vi "Global Event Filter Example - Filter From Subscriber.vi"() -> ()   [LabVIEW 2017]
uses:
  user.lib/_NEVSTOP/Communicable State Machine(CSM)/_Support/Typedef/_CSM_GlobalLog Filter Rules - v1.0.ctl
  user.lib/_NEVSTOP/Communicable State Machine(CSM)/_Support/Typedef/_CSM_GlobalLog_MSG_TYPE.ctl
  user.lib/_NEVSTOP/Communicable State Machine(CSM)/_Support/Typedef/_CSM_GlobalLog_STATE_TYPE.ctl
  user.lib/_NEVSTOP/Communicable State Machine(CSM)/_Support/Typedef/_CSM_GlobalLog_MSG.ctl
  user.lib/_NEVSTOP/Communicable State Machine(CSM)/_Support/Typedef/_CSM_Response Source Message.ctl
  user.lib/_NEVSTOP/Communicable State Machine(CSM)/_Support/GlobalEvent/Gevt-ThreadQueueName.vi
  user.lib/_NEVSTOP/Communicable State Machine(CSM)/_Support/GlobalEvent/GEvt-Filter Global Log - v1.0.vi
  user.lib/_NEVSTOP/Communicable State Machine(CSM)/Communicable State Machine.lvlib
panel:
  in  "Rules-v1":T1={"Global"={"CSM"=["Module2"], "LogType"=[], "State"=[], "StateType"=[]}, "CSM"={"LogType"=[{"CSM"="Module1", "LogType"=enum."State Change"}], "State"=[{"CSM"="Module3", "State"=""}], "StateType"=[]}}
  out "State History":string="[2024/08/26 12:22:52.862]  [State Change] Module2 | DoSth: Check If Greater than 0.5\r[2024/08/26 12:22:52.861]  [State Change] Module4 | DoSth: Check If Greater than 0.5\r[2024/08/26 12:22:52.859]  [State Change] Module1 | DoSth: Check If Greater than 0.5\r[2024/08/26 12:22:52.856]  [State Change] Module3 | DoSth: Check If Greater than 0.5\r[2024/08/26 12:22:51.861]  [State Change] Module2 | DoSth: Check If Greater than 0.5\r[2024/08/26 12:22:51.859]  [State Change] Module4 | DoSth: Check If Greater than 0.5\r[2024/08/26 12:22:51.857]  [State Change] Module1 | DoSth: Check If Greater than 0.5\r[2024/08/26 12:22:51.855]  [State Change] Module3 | DoSth: Check If Greater than 0.5\r[2024/08/26 12:22:50.861]  [State Change] Module2 | DoSth: Check If Greater than 0.5\r[2024/08/26 12:22:50.859]  [State Change] Module4 | DoSth: Check If Greater than 0.5\r[2024/08/26 12:22:50.857]  [State Change] Module1 | DoSth: Check If Greater than 0.5\r[2024/08/26 12:22:50.855]  [State Change] Module3 | DoSth: Check If Greater than 0.5\r[2024/08/26 12:22:49.861]  [State Change] Module2 | DoSth: Check If Greater than 0.5\r[2024/08/26 12:22:49.858]  [State Change] Module4 | DoSth: Check If Greater than 0.5\r[2024/08/26 12:22:49.856]  [State Change] Module1 | DoSth: Check If Greater than 0.5\r[2024/08/26 12:22:49.854]  [State Change] Module3 | DoSth: Check If Greater than 0.5\r[2024/08/26 12:22:48.858]  [State Change] Module2 | DoSth: Check If Greater than 0.5\r[2024/08/26 12:22:48.858]  [State Change] Module4 | DoSth: Check If Greater than 0.5\r[2024/08/26 12:22:48.856]  [State Change] Module1 | DoSth: Check If Greater than 0.5\r[2024/08/26 12:22:48.854]  [State Change] Module3 | DoSth: Check If Greater than 0.5\r[2024/08/26 12:22:43.853]  [Status] Module2 | Status Changed >> 0.966426\r[2024/08/26 12:22:43.853]  [Status] Module2 | Another Status\r[2024/08/26 12:22:43.851]  [Status] Module4 | Status Changed >> 0.587309\r[2024/08/26 12:22:43.851]  [Status] Module4 | Another Status\r[2024/08/26 12:22:43.851]  [Status] Module3 | Status Changed >> 0.609550\r[2024/08/26 12:22:43.850]  [Status] Module3 | Another Status\r[2024/08/26 12:22:42.853]  [Status] Module2 | Status Changed >> 0.657896\r[2024/08/26 12:22:42.853]  [Status] Module2 | Another Status\r[2024/08/26 12:22:41.853]  [Status] Module1 | Status Changed >> 0.612353\r[2024/08/26 12:22:41.853]  [Status] Module1 | Another Status\r[2024/08/26 12:22:41.850]  [Status] Module3 | Status Changed >> 0.903353\r[2024/08/26 12:22:41.850]  [Status] Module4 | Status Changed >> 0.752577\r[2024/08/26 12:22:41.850]  [Status] Module3 | Another Status\r[2024/08/26 12:22:41.850]  [Status] Module4 | Another Status\r[2024/08/26 12:22:40.853]  [Status] Module1 | Status Changed >> 0.793800\r[2024/08/26 12:22:40.853]  [Status] Module2 | Status Changed >> 0.661958\r[2024/08/26 12:22:40.853]  [Status] Module1 | Another Status\r[2024/08/26 12:22:40.853]  [Status] Module2 | Another Status\r[2024/08/26 12:22:40.850]  [Status] Module4 | Status Changed >> 0.812931\r[2024/08/26 12:22:40.850]  [Status] Module4 | Another Status\r[2024/08/26 12:22:39.853]  [Status] Module1 | Status Changed >> 0.533631\r[2024/08/26 12:22:39.853]  [Status] Module2 | Status Changed >> 0.784890\r[2024/08/26 12:22:39.853]  [Status] Module1 | Another Status\r[2024/08/26 12:22:39.853]  [Status] Module2 | Another Status\r[2024/08/26 12:22:38.853]  [Status] Module2 | Status Changed >> 0.650802\r[2024/08/26 12:22:38.852]  [Status] Module2 | Another Status\r[2024/08/26 12:22:37.848]  [Status] Module4 | Status Changed >> 0.644286\r[2024/08/26 12:22:37.848]  [Status] Module4 | Another Status\r[2024/08/26 12:22:36.851]  [Status] Module1 | Status Changed >> 0.717178\r[2024/08/26 12:22:36.851]  [Status] Module1 | Another Status\r[2024/08/26 12:22:36.850]  [Status] Module2 | Status Changed >> 0.778432\r[2024/08/26 12:22:36.850]  [Status] Module2 | Another Status\r[2024/08/26 12:22:36.848]  [Status] Module3 | Status Changed >> 0.926927\r[2024/08/26 12:22:36.847]  [Status] Module4 | Status Changed >> 0.767567\r[2024/08/26 12:22:36.847]  [Status] Module3 | Another Status\r[2024/08/26 12:22:36.847]  [Status] Module4 | Another Status\r[2024/08/26 12:22:35.846]  [Status] Module3 | Status Changed >> 0.714868\r[2024/08/26 12:22:35.846]  [Status] Module3 | Another Status\r[2024/08/26 12:22:34.846]  [Status] Module4 | Status Changed >> 0.978272\r[2024/08/26 12:22:34.846]  [Status] Module4 | Another Status\r[2024/08/26 12:22:33.850]  [Status] Module1 | Status Changed >> 0.724023\r[2024/08/26 12:22:33.850]  [Status] Module1 | Another Status\r[2024/08/26 12:22:33.845]  [Status] Module4 | Status Changed >> 0.761429\r[2024/08/26 12:22:33.845]  [Status] Module3 | Status Changed >> 0.870243\r[2024/08/26 12:22:33.845]  [Status] Module4 | Another Status\r[2024/08/26 12:22:33.845]  [Status] Module3 | Another Status\r[2024/08/26 12:22:31.847]  [Status] Module2 | Status Changed >> 0.716248\r[2024/08/26 12:22:31.847]  [Status] Module2 | Another Status\r[2024/08/26 12:22:31.845]  [Status] Module3 | Status Changed >> 0.746803\r[2024/08/26 12:22:31.845]  [Status] Module3 | Another Status\r[2024/08/26 12:22:30.844]  [Status] Module4 | Status Changed >> 0.503995\r[2024/08/26 12:22:30.844]  [Status] Module3 | Status Changed >> 0.761523\r[2024/08/26 12:22:30.844]  [Status] Module4 | Another Status\r[2024/08/26 12:22:30.844]  [Status] Module3 | Another Status\r[2024/08/26 12:22:29.848]  [Status] Module1 | Status Changed >> 0.618764\r[2024/08/26 12:22:29.848]  [Status] Module1 | Another Status\r[2024/08/26 12:22:29.844]  [Status] Module3 | Status Changed >> 0.963232\r[2024/08/26 12:22:29.844]  [Status] Module3 | Another Status\r[2024/08/26 12:22:28.846]  [Status] Module2 | Status Changed >> 0.965763\r[2024/08/26 12:22:28.846]  [Status] Module2 | Another Status\r[2024/08/26 12:22:28.844]  [Status] Module4 | Status Changed >> 0.926638\r[2024/08/26 12:22:28.844]  [Status] Module3 | Status Changed >> 0.912527\r[2024/08/26 12:22:28.844]  [Status] Module3 | Another Status\r[2024/08/26 12:22:28.844]  [Status] Module4 | Another Status\r[2024/08/26 12:22:27.845]  [State Change] Module1 | DoSth: Check If Greater than 0.5\r[2024/08/26 12:22:27.845]  [State Change] Module2 | DoSth: Check If Greater than 0.5\r[2024/08/26 12:22:27.844]  [State Change] Module3 | DoSth: Check If Greater than 0.5\r[2024/08/26 12:22:27.844]  [State Change] Module4 | DoSth: Check If Greater than 0.5\r[2024/08/26 12:22:26.845]  [State Change] Module2 | DoSth: Check If Greater than 0.5\r[2024/08/26 12:22:26.845]  [State Change] Module1 | DoSth: Check If Greater than 0.5\r[2024/08/26 12:22:26.844]  [State Change] Module3 | DoSth: Check If Greater than 0.5\r[2024/08/26 12:22:26.844]  [State Change] Module4 | DoSth: Check If Greater than 0.5\r[2024/08/26 12:22:25.844]  [State Change] Module1 | DoSth: Check If Greater than 0.5\r[2024/08/26 12:22:25.844]  [State Change] Module2 | DoSth: Check If Greater than 0.5\r[2024/08/26 12:22:25.842]  [State Change] Module4 | DoSth: Check If Greater than 0.5\r[2024/08/26 12:22:25.842]  [State Change] Module3 | DoSth: Check If Greater than 0.5\r[2024/08/26 12:22:24.845]  [State Change] Module1 | DoSth: Check If Greater than 0.5\r[2024/08/26 12:22:24.845]  [State Change] Module2 | DoSth: Check If Greater than 0.5\r[2024/08/26 12:22:24.842]  [State Change] Module4 | DoSth: Check If Greater than 0.5\r[2024/08/26 12:22:24.842]  [State Change] Module3 | DoSth: Check If Greater than 0.5\r[2024/08/26 12:22:23.844]  [State Change] Module1 | DoSth: Check If Greater than 0.5\r[2024/08/26 12:22:23.841]  [State Change] Module4 | DoSth: Check If Greater than 0.5\r[2024/08/26 12:22:23.841]  [State Change] Module2 | DoSth: Check If Greater than 0.5\r[2024/08/26 12:22:23.841]  [State Change] Module3 | DoSth: Check If Greater than 0.5\r[2024/08/26 12:22:22.844]  [State Change] Module1 | DoSth: Check If Greater than 0.5\r[2024/08/26 12:22:22.840]  [State Change] Module4 | DoSth: Check If Greater than 0.5\r[2024/08/26 12:22:22.840]  [State Change] Module3 | DoSth: Check If Greater than 0.5\r[2024/08/26 12:22:22.840]  [State Change] Module2 | DoSth: Check If Greater than 0.5\r[2024/08/26 12:22:21.843]  [State Change] Module1 | DoSth: Check If Greater than 0.5\r[2024/08/26 12:22:21.840]  [State Change] Module4 | DoSth: Check If Greater than 0.5\r[2024/08/26 12:22:21.839]  [State Change] Module3 | DoSth: Check If Greater than 0.5\r[2024/08/26 12:22:21.838]  [State Change] Module2 | DoSth: Check If Greater than 0.5\r[2024/08/26 12:22:20.842]  [State Change] Module1 | DoSth: Check If Greater than 0.5\r[2024/08/26 12:22:20.840]  [Status] Module4 | Status Changed >> 0.842847\r[2024/08/26 12:22:20.840]  [Status] Module4 | Another Status\r[2024/08/26 12:22:20.839]  [State Change] Module3 | DoSth: Check If Greater than 0.5\r[2024/08/26 12:22:20.839]  [State Change] Module4 | DoSth: Check If Greater than 0.5\r[2024/08/26 12:22:20.838]  [Status] Module2 | Status Changed >> 0.886493\r[2024/08/26 12:22:20.838]  [Status] Module2 | Another Status\r[2024/08/26 12:22:20.838]  [State Change] Module2 | DoSth: Check If Greater than 0.5\r[2024/08/26 12:22:19.842]  [Status] Module1 | Status Changed >> 0.854895\r[2024/08/26 12:22:19.842]  [Status] Module1 | Another Status\r[2024/08/26 12:22:19.842]  [State Change] Module1 | DoSth: Check If Greater than 0.5\r[2024/08/26 12:22:19.840]  [Status] Module4 | Status Changed >> 0.878715\r[2024/08/26 12:22:19.839]  [Status] Module4 | Another Status\r[2024/08/26 12:22:19.839]  [State Change] Module4 | DoSth: Check If Greater than 0.5\r[2024/08/26 12:22:19.839]  [Status] Module3 | Status Changed >> 0.716873\r[2024/08/26 12:22:19.839]  [Status] Module3 | Another Status\r[2024/08/26 12:22:19.838]  [State Change] Module3 | DoSth: Check If Greater than 0.5\r[2024/08/26 12:22:19.838]  [State Change] Module2 | DoSth: Check If Greater than 0.5\r[2024/08/26 12:22:18.841]  [Status] Module1 | Status Changed >> 0.566399\r[2024/08/26 12:22:18.840]  [Status] Module1 | Another Status\r[2024/08/26 12:22:18.840]  [State Change] Module1 | DoSth: Check If Greater than 0.5\r[2024/08/26 12:22:18.839]  [State Change] Module4 | DoSth: Check If Greater than 0.5\r[2024/08/26 12:22:18.838]  [Status] Module2 | Status Changed >> 0.734045\r[2024/08/26 12:22:18.838]  [Status] Module2 | Another Status\r[2024/08/26 12:22:18.838]  [State Change] Module2 | DoSth: Check If Greater than 0.5\r[2024/08/26 12:22:18.838]  [State Change] Module3 | DoSth: Check If Greater than 0.5\r[2024/08/26 12:22:17.840]  [Status] Module1 | Status Changed >> 0.702477\r[2024/08/26 12:22:17.840]  [Status] Module1 | Another Status\r[2024/08/26 12:22:17.840]  [State Change] Module1 | DoSth: Check If Greater than 0.5\r[2024/08/26 12:22:17.839]  [Status] Module4 | Status Changed >> 0.500518\r[2024/08/26 12:22:17.839]  [Status] Module4 | Another Status\r[2024/08/26 12:22:17.839]  [State Change] Module4 | DoSth: Check If Greater than 0.5\r[2024/08/26 12:22:17.837]  [Status] Module3 | Status Changed >> 0.815805\r[2024/08/26 12:22:17.837]  [Status] Module3 | Another Status\r[2024/08/26 12:22:17.837]  [State Change] Module2 | DoSth: Check If Greater than 0.5\r[2024/08/26 12:22:17.837]  [State Change] Module3 | DoSth: Check If Greater than 0.5\r[2024/08/26 12:22:16.841]  [State Change] Module1 | DoSth: Check If Greater than 0.5\r[2024/08/26 12:22:16.839]  [State Change] Module4 | DoSth: Check If Greater than 0.5\r[2024/08/26 12:22:16.838]  [Status] Module2 | Status Changed >> 0.992609\r[2024/08/26 12:22:16.838]  [Status] Module2 | Another Status\r[2024/08/26 12:22:16.837]  [State Change] Module2 | DoSth: Check If Greater than 0.5\r[2024/08/26 12:22:16.837]  [State Change] Module3 | DoSth: Check If Greater than 0.5\r[2024/08/26 12:22:15.840]  [Status] Module1 | Status Changed >> 0.906384\r[2024/08/26 12:22:15.840]  [Status] Module1 | Another Status\r[2024/08/26 12:22:15.839]  [State Change] Module1 | DoSth: Check If Greater than 0.5\r[2024/08/26 12:22:15.839]  [State Change] Module4 | DoSth: Check If Greater than 0.5\r[2024/08/26 12:22:15.837]  [Status] Module3 | Status Changed >> 0.571918\r[2024/08/26 12:22:15.837]  [Status] Module3 | Another Status\r[2024/08/26 12:22:15.837]  [State Change] Module2 | DoSth: Check If Greater than 0.5\r[2024/08/26 12:22:15.837]  [State Change] Module3 | DoSth: Check If Greater than 0.5\r[2024/08/26 12:22:14.839]  [Status] Module4 | Status Changed >> 0.664332\r[2024/08/26 12:22:14.839]  [Status] Module4 | Another Status\r[2024/08/26 12:22:14.838]  [State Change] Module4 | DoSth: Check If Greater than 0.5\r[2024/08/26 12:22:14.837]  [Status] Module3 | Status Changed >> 0.894203\r[2024/08/26 12:22:14.837]  [Status] Module1 | Status Changed >> 0.623354\r[2024/08/26 12:22:14.837]  [Status] Module3 | Another Status\r[2024/08/26 12:22:14.837]  [Status] Module2 | Status Changed >> 0.893231\r[2024/08/26 12:22:14.837]  [Status] Module1 | Another Status\r[2024/08/26 12:22:14.836]  [Status] Module2 | Another Status\r[2024/08/26 12:22:14.836]  [State Change] Module3 | DoSth: Check If Greater than 0.5\r[2024/08/26 12:22:14.836]  [State Change] Module1 | DoSth: Check If Greater than 0.5\r[2024/08/26 12:22:14.835]  [State Change] Module2 | DoSth: Check If Greater than 0.5\r[2024/08/26 12:22:13.838]  [Status] Module4 | Status Changed >> 0.758699\r[2024/08/26 12:22:13.838]  [Status] Module4 | Another Status\r[2024/08/26 12:22:13.837]  [State Change] Module4 | DoSth: Check If Greater than 0.5\r[2024/08/26 12:22:13.836]  [State Change] Module3 | DoSth: Check If Greater than 0.5\r[2024/08/26 12:22:13.835]  [State Change] Module1 | DoSth: Check If Greater than 0.5\r[2024/08/26 12:22:13.835]  [Status] Module2 | Status Changed >> 0.869280\r[2024/08/26 12:22:13.835]  [Status] Module2 | Another Status\r[2024/08/26 12:22:13.834]  [State Change] Module2 | DoSth: Check If Greater than 0.5\r[2024/08/26 12:22:12.836]  [State Change] Module4 | DoSth: Check If Greater than 0.5\r[2024/08/26 12:22:12.835]  [Status] Module1 | Status Changed >> 0.612032\r[2024/08/26 12:22:12.835]  [Status] Module3 | Status Changed >> 0.560119\r[2024/08/26 12:22:12.835]  [Status] Module1 | Another Status\r[2024/08/26 12:22:12.835]  [Status] Module3 | Another Status\r[2024/08/26 12:22:12.835]  [State Change] Module3 | DoSth: Check If Greater than 0.5\r[2024/08/26 12:22:12.835]  [State Change] Module1 | DoSth: Check If Greater than 0.5\r[2024/08/26 12:22:12.833]  [Status] Module2 | Status Changed >> 0.555002\r[2024/08/26 12:22:12.833]  [Status] Module2 | Another Status\r[2024/08/26 12:22:12.833]  [State Change] Module2 | DoSth: Check If Greater than 0.5\r[2024/08/26 12:22:11.837]  [Status] Module4 | Status Changed >> 0.724141\r[2024/08/26 12:22:11.836]  [Status] Module4 | Another Status\r[2024/08/26 12:22:11.836]  [State Change] Module4 | DoSth: Check If Greater than 0.5\r[2024/08/26 12:22:11.835]  [Status] Module1 | Status Changed >> 0.922671\r[2024/08/26 12:22:11.835]  [Status] Module3 | Status Changed >> 0.837689\r[2024/08/26 12:22:11.835]  [Status] Module1 | Another Status\r[2024/08/26 12:22:11.835]  [Status] Module3 | Another Status\r[2024/08/26 12:22:11.834]  [State Change] Module1 | DoSth: Check If Greater than 0.5\r[2024/08/26 12:22:11.834]  [State Change] Module3 | DoSth: Check If Greater than 0.5\r[2024/08/26 12:22:11.833]  [Status] Module2 | Status Changed >> 0.556129\r[2024/08/26 12:22:11.833]  [Status] Module2 | Another Status\r[2024/08/26 12:22:11.832]  [State Change] Module2 | DoSth: Check If Greater than 0.5\r[2024/08/26 12:22:10.836]  [Status] Module4 | Status Changed >> 0.659149\r[2024/08/26 12:22:10.835]  [Status] Module3 | Status Changed >> 0.524146\r[2024/08/26 12:22:10.835]  [Status] Module1 | Status Changed >> 0.794492\r[2024/08/26 12:22:10.835]  [Status] Module4 | Another Status\r[2024/08/26 12:22:10.835]  [Status] Module3 | Another Status\r[2024/08/26 12:22:10.834]  [Status] Module1 | Another Status\r[2024/08/26 12:22:10.834]  [State Change] Module4 | DoSth: Check If Greater than 0.5\r[2024/08/26 12:22:10.834]  [State Change] Module3 | DoSth: Check If Greater than 0.5\r[2024/08/26 12:22:10.833]  [State Change] Module1 | DoSth: Check If Greater than 0.5\r[2024/08/26 12:22:10.832]  [Status] Module2 | Status Changed >> 0.893687\r[2024/08/26 12:22:10.832]  [Status] Module2 | Another Status\r[2024/08/26 12:22:10.831]  [State Change] Module2 | DoSth: Check If Greater than 0.5\r[2024/08/26 12:22:09.833]  [Status] Module4 | Status Changed >> 0.649413\r[2024/08/26 12:22:09.833]  [Status] Module4 | Another Status\r[2024/08/26 12:22:09.833]  [State Change] Module3 | DoSth: Check If Greater than 0.5\r[2024/08/26 12:22:09.833]  [State Change] Module4 | DoSth: Check If Greater than 0.5\r[2024/08/26 12:22:09.833]  [State Change] Module1 | DoSth: Check If Greater than 0.5\r[2024/08/26 12:22:09.831]  [State Change] Module2 | DoSth: Check If Greater than 0.5\r[2024/08/26 12:22:08.833]  [Status] Module4 | Status Changed >> 0.853627\r[2024/08/26 12:22:08.833]  [Status] Module4 | Another Status\r[2024/08/26 12:22:08.833]  [State Change] Module1 | DoSth: Check If Greater than 0.5\r[2024/08/26 12:22:08.833]  [State Change] Module3 | DoSth: Check If Greater than 0.5\r[2024/08/26 12:22:08.832]  [State Change] Module4 | DoSth: Check If Greater than 0.5\r[2024/08/26 12:22:08.830]  [State Change] Module2 | DoSth: Check If Greater than 0.5\r[2024/08/26 12:22:07.831]  [Status] Module4 | Status Changed >> 0.944577\r[2024/08/26 12:22:07.831]  [Status] Module3 | Status Changed >> 0.936581\r[2024/08/26 12:22:07.831]  [Status] Module4 | Another Status\r[2024/08/26 12:22:07.831]  [Status] Module3 | Another Status\r[2024/08/26 12:22:07.831]  [State Change] Module4 | DoSth: Check If Greater than 0.5\r[2024/08/26 12:22:07.831]  [State Change] Module3 | DoSth: Check If Greater than 0.5\r[2024/08/26 12:22:07.831]  [State Change] Module1 | DoSth: Check If Greater than 0.5\r[2024/08/26 12:22:07.830]  [Status] Module2 | Status Changed >> 0.819259\r[2024/08/26 12:22:07.829]  [Status] Module2 | Another Status\r[2024/08/26 12:22:07.829]  [State Change] Module2 | DoSth: Check If Greater than 0.5\r[2024/08/26 12:22:06.831]  [Status] Module3 | Status Changed >> 0.883823\r[2024/08/26 12:22:06.831]  [Status] Module3 | Another Status\r[2024/08/26 12:22:06.831]  [State Change] Module3 | DoSth: Check If Greater than 0.5\r[2024/08/26 12:22:06.831]  [State Change] Module4 | DoSth: Check If Greater than 0.5\r[2024/08/26 12:22:06.831]  [State Change] Module1 | DoSth: Check If Greater than 0.5\r[2024/08/26 12:22:06.829]  [Status] Module2 | Status Changed >> 0.641694\r[2024/08/26 12:22:06.829]  [Status] Module2 | Another Status\r[2024/08/26 12:22:06.829]  [State Change] Module2 | DoSth: Check If Greater than 0.5\r[2024/08/26 12:22:05.831]  [Status] Module4 | Status Changed >> 0.612309\r[2024/08/26 12:22:05.831]  [Status] Module4 | Another Status\r[2024/08/26 12:22:05.831]  [State Change] Module4 | DoSth: Check If Greater than 0.5\r[2024/08/26 12:22:05.831]  [State Change] Module1 | DoSth: Check If Greater than 0.5\r[2024/08/26 12:22:05.831]  [State Change] Module3 | DoSth: Check If Greater than 0.5\r[2024/08/26 12:22:05.829]  [Status] Module2 | Status Changed >> 0.689023\r[2024/08/26 12:22:05.829]  [Status] Module2 | Another Status\r[2024/08/26 12:22:05.829]  [State Change] Module2 | DoSth: Check If Greater than 0.5\r[2024/08/26 12:22:04.832]  [Status] Module1 | Status Changed >> 0.574610\r[2024/08/26 12:22:04.832]  [Status] Module4 | Status Changed >> 0.669847\r[2024/08/26 12:22:04.832]  [Status] Module1 | Another Status\r[2024/08/26 12:22:04.832]  [Status] Module4 | Another Status\r[2024/08/26 12:22:04.832]  [State Change] Module4 | DoSth: Check If Greater than 0.5\r[2024/08/26 12:22:04.831]  [State Change] Module1 | DoSth: Check If Greater than 0.5\r[2024/08/26 12:22:04.831]  [State Change] Module3 | DoSth: Check If Greater than 0.5\r[2024/08/26 12:22:04.829]  [State Change] Module2 | DoSth: Check If Greater than 0.5\r[2024/08/26 12:22:03.831]  [State Change] Module1 | \r[2024/08/26 12:22:03.830]  [State Change] Module1 | DoSth: Check If Greater than 0.5\r[2024/08/26 12:22:03.830]  [State Change] Module4 | \r[2024/08/26 12:22:03.830]  [Status] Module4 | Status Changed >> 0.753361\r[2024/08/26 12:22:03.830]  [Status] Module4 | Another Status\r[2024/08/26 12:22:03.830]  [State Change] Module3 | \r[2024/08/26 12:22:03.830]  [State Change] Module2 | \r[2024/08/26 12:22:03.830]  [State Change] Module3 | DoSth: Check If Greater than 0.5\r[2024/08/26 12:22:03.830]  [State Change] Module4 | DoSth: Check If Greater than 0.5\r[2024/08/26 12:22:03.829]  [State Change] Module2 | DoSth: Check If Greater than 0.5\r[2024/08/26 12:22:02.830]  [State Change] Module1 | \r[2024/08/26 12:22:02.829]  [State Change] Module4 | \r[2024/08/26 12:22:02.829]  [Status] Module4 | Status Changed >> 0.861013\r[2024/08/26 12:22:02.829]  [Status] Module4 | Another Status\r[2024/08/26 12:22:02.829]  [State Change] Module2 | \r[2024/08/26 12:22:02.829]  [Status] Module2 | Status Changed >> 0.737404\r[2024/08/26 12:22:02.829]  [State Change] Module4 | DoSth: Check If Greater than 0.5\r[2024/08/26 12:22:02.829]  [Status] Module1 | Status Changed >> 0.953716\r[2024/08/26 12:22:02.829]  [Status] Module2 | Another Status\r[2024/08/26 12:22:02.828]  [State Change] Module3 | \r[2024/08/26 12:22:02.828]  [Status] Module1 | Another Status\r[2024/08/26 12:22:02.828]  [State Change] Module3 | DoSth: Check If Greater than 0.5\r[2024/08/26 12:22:02.828]  [State Change] Module2 | DoSth: Check If Greater than 0.5\r[2024/08/26 12:22:02.828]  [State Change] Module1 | DoSth: Check If Greater than 0.5\r[2024/08/26 12:22:01.828]  [State Change] Module4 | \r[2024/08/26 12:22:01.828]  [State Change] Module4 | DoSth: Check If Greater than 0.5\r[2024/08/26 12:22:01.827]  [State Change] Module1 | \r[2024/08/26 12:22:01.827]  [State Change] Module3 | \r[2024/08/26 12:22:01.826]  [State Change] Module3 | DoSth: Check If Greater than 0.5\r[2024/08/26 12:22:01.826]  [State Change] Module2 | \r[2024/08/26 12:22:01.826]  [Status] Module2 | Status Changed >> 0.699250\r[2024/08/26 12:22:01.826]  [Status] Module1 | Status Changed >> 0.570538\r[2024/08/26 12:22:01.826]  [Status] Module2 | Another Status\r[2024/08/26 12:22:01.825]  [Status] Module1 | Another Status\r[2024/08/26 12:22:01.825]  [State Change] Module2 | DoSth: Check If Greater than 0.5\r[2024/08/26 12:22:01.825]  [State Change] Module1 | DoSth: Check If Greater than 0.5\r[2024/08/26 12:22:00.829]  [State Change] Module4 | \r[2024/08/26 12:22:00.829]  [Status] Module4 | Status Changed >> 0.931921\r[2024/08/26 12:22:00.827]  [State Change] Module3 | \r[2024/08/26 12:22:00.827]  [Status] Module3 | Status Changed >> 0.915043\r[2024/08/26 12:22:00.827]  [State Change] Module2 | \r[2024/08/26 12:22:00.826]  [State Change] Module1 | \r[2024/08/26 12:22:00.826]  [Status] Module2 | Status Changed >> 0.884983\r[2024/08/26 12:22:00.826]  [Status] Module1 | Status Changed >> 0.542614\r[2024/08/26 12:22:00.826]  [Status] Module3 | Another Status\r[2024/08/26 12:22:00.826]  [Status] Module4 | Another Status\r[2024/08/26 12:22:00.826]  [Status] Module2 | Another Status\r[2024/08/26 12:22:00.826]  [Status] Module1 | Another Status\r[2024/08/26 12:22:00.825]  [State Change] Module3 | DoSth: Check If Greater than 0.5\r[2024/08/26 12:22:00.825]  [State Change] Module2 | DoSth: Check If Greater than 0.5\r[2024/08/26 12:22:00.825]  [State Change] Module4 | DoSth: Check If Greater than 0.5\r[2024/08/26 12:22:00.824]  [State Change] Module1 | DoSth: Check If Greater than 0.5\r[2024/08/26 12:21:59.824]  [State Change] Module3 | \r[2024/08/26 12:21:59.824]  [State Change] Module4 | \r[2024/08/26 12:21:59.824]  [Status] Module3 | Status Changed >> 0.811042\r[2024/08/26 12:21:59.824]  [Status] Module4 | Status Changed >> 0.721776\r[2024/08/26 12:21:59.824]  [Status] Module3 | Another Status\r[2024/08/26 12:21:59.824]  [Status] Module4 | Another Status\r[2024/08/26 12:21:59.824]  [State Change] Module1 | \r[2024/08/26 12:21:59.824]  [State Change] Module2 | \r[2024/08/26 12:21:59.824]  [State Change] Module3 | DoSth: Check If Greater than 0.5\r[2024/08/26 12:21:59.824]  [State Change] Module1 | DoSth: Check If Greater than 0.5\r[2024/08/26 12:21:59.824]  [State Change] Module2 | DoSth: Check If Greater than 0.5\r[2024/08/26 12:21:59.824]  [State Change] Module4 | DoSth: Check If Greater than 0.5\r[2024/08/26 12:21:58.825]  [State Change] Module1 | \r[2024/08/26 12:21:58.825]  [State Change] Module3 | \r[2024/08/26 12:21:58.825]  [Status] Module1 | Status Changed >> 0.921429\r[2024/08/26 12:21:58.825]  [Status] Module3 | Status Changed >> 0.988557\r[2024/08/26 12:21:58.825]  [Status] Module1 | Another Status\r[2024/08/26 12:21:58.825]  [State Change] Module2 | \r[2024/08/26 12:21:58.825]  [Status] Module3 | Another Status\r[2024/08/26 12:21:58.825]  [State Change] Module4 | \r[2024/08/26 12:21:58.825]  [State Change] Module1 | DoSth: Check If Greater than 0.5\r[2024/08/26 12:21:58.824]  [State Change] Module2 | DoSth: Check If Greater than 0.5\r[2024/08/26 12:21:58.824]  [State Change] Module4 | DoSth: Check If Greater than 0.5\r[2024/08/26 12:21:58.824]  [State Change] Module3 | DoSth: Check If Greater than 0.5\r[2024/08/26 12:21:57.825]  [State Change] Module3 | \r[2024/08/26 12:21:57.825]  [State Change] Module4 | \r[2024/08/26 12:21:57.825]  [Status] Module3 | Status Changed >> 0.790884\r[2024/08/26 12:21:57.825]  [State Change] Module4 | DoSth: Check If Greater than 0.5\r[2024/08/26 12:21:57.825]  [State Change] Module1 | \r[2024/08/26 12:21:57.825]  [Status] Module1 | Status Changed >> 0.712844\r[2024/08/26 12:21:57.825]  [Status] Module3 | Another Status\r[2024/08/26 12:21:57.825]  [Status] Module1 | Another Status\r[2024/08/26 12:21:57.824]  [State Change] Module2 | \r[2024/08/26 12:21:57.824]  [State Change] Module2 | DoSth: Check If Greater than 0.5\r[2024/08/26 12:21:57.824]  [State Change] Module3 | DoSth: Check If Greater than 0.5\r[2024/08/26 12:21:57.823]  [State Change] Module1 | DoSth: Check If Greater than 0.5\r[2024/08/26 12:21:56.824]  [State Change] Module4 | \r[2024/08/26 12:21:56.824]  [Status] Module4 | Status Changed >> 0.874396\r[2024/08/26 12:21:56.824]  [Status] Module4 | Another Status\r[2024/08/26 12:21:56.824]  [State Change] Module1 | \r[2024/08/26 12:21:56.824]  [State Change] Module2 | \r[2024/08/26 12:21:56.824]  [State Change] Module4 | DoSth: Check If Greater than 0.5\r[2024/08/26 12:21:56.823]  [State Change] Module1 | DoSth: Check If Greater than 0.5\r[2024/08/26 12:21:56.823]  [State Change] Module2 | DoSth: Check If Greater than 0.5\r[2024/08/26 12:21:56.823]  [State Change] Module3 | \r[2024/08/26 12:21:56.822]  [State Change] Module3 | DoSth: Check If Greater than 0.5\r[2024/08/26 12:21:55.824]  [State Change] Module4 | \r[2024/08/26 12:21:55.824]  [State Change] Module1 | \r[2024/08/26 12:21:55.824]  [Status] Module4 | Status Changed >> 0.636618\r[2024/08/26 12:21:55.824]  [Status] Module1 | Status Changed >> 0.791454\r[2024/08/26 12:21:55.824]  [State Change] Module2 | \r[2024/08/26 12:21:55.823]  [State Change] Module2 | DoSth: Check If Greater than 0.5\r[2024/08/26 12:21:55.823]  [Status] Module4 | Another Status\r[2024/08/26 12:21:55.823]  [Status] Module1 | Another Status\r[2024/08/26 12:21:55.823]  [State Change] Module3 | \r[2024/08/26 12:21:55.823]  [State Change] Module3 | DoSth: Check If Greater than 0.5\r[2024/08/26 12:21:55.822]  [State Change] Module4 | DoSth: Check If Greater than 0.5\r[2024/08/26 12:21:55.822]  [State Change] Module1 | DoSth: Check If Greater than 0.5\r[2024/08/26 12:21:54.822]  [State Change] Module2 | \r[2024/08/26 12:21:54.822]  [Status] Module2 | Status Changed >> 0.861404\r[2024/08/26 12:21:54.822]  [Status] Module2 | Another Status\r[2024/08/26 12:21:54.822]  [State Change] Module1 | \r[2024/08/26 12:21:54.822]  [State Change] Module3 | \r[2024/08/26 12:21:54.821]  [State Change] Module4 | \r[2024/08/26 12:21:54.821]  [State Change] Module1 | DoSth: Check If Greater than 0.5\r[2024/08/26 12:21:54.821]  [State Change] Module2 | DoSth: Check If Greater than 0.5\r[2024/08/26 12:21:54.821]  [State Change] Module3 | DoSth: Check If Greater than 0.5\r[2024/08/26 12:21:54.821]  [State Change] Module4 | DoSth: Check If Greater than 0.5\r[2024/08/26 12:21:53.820]  [State Change] Module4 | \r[2024/08/26 12:21:53.820]  [State Change] Module3 | \r[2024/08/26 12:21:53.820]  [State Change] Module2 | \r[2024/08/26 12:21:53.820]  [State Change] Module1 | \r[2024/08/26 12:21:53.820]  [Status] Module4 | Check Started\r[2024/08/26 12:21:53.820]  [State Change] Module4 | API: Start(Complete) <- -PostMsgAPICFE158F76420\r[2024/08/26 12:21:53.820]  [Status] Module3 | Check Started\r[2024/08/26 12:21:53.820]  [Status] Module2 | Check Started\r[2024/08/26 12:21:53.820]  [Status] Module1 | Check Started\r[2024/08/26 12:21:53.819]  [State Change] Module3 | API: Start(Complete) <- -PostMsgAPICFE158F76420\r[2024/08/26 12:21:53.819]  [State Change] Module2 | API: Start(Complete) <- -PostMsgAPICFE158F76420\r[2024/08/26 12:21:53.819]  [State Change] Module4 | API: Start <- -PostMsgAPICFE158F76420\r[2024/08/26 12:21:53.819]  [State Change] Module1 | API: Start(Complete) <- -PostMsgAPICFE158F76420\r[2024/08/26 12:21:53.819]  [State Change] Module3 | API: Start <- -PostMsgAPICFE158F76420\r[2024/08/26 12:21:53.819]  [State Change] Module2 | API: Start <- -PostMsgAPICFE158F76420\r[2024/08/26 12:21:53.818]  [State Change] Module1 | API: Start <- -PostMsgAPICFE158F76420\r"
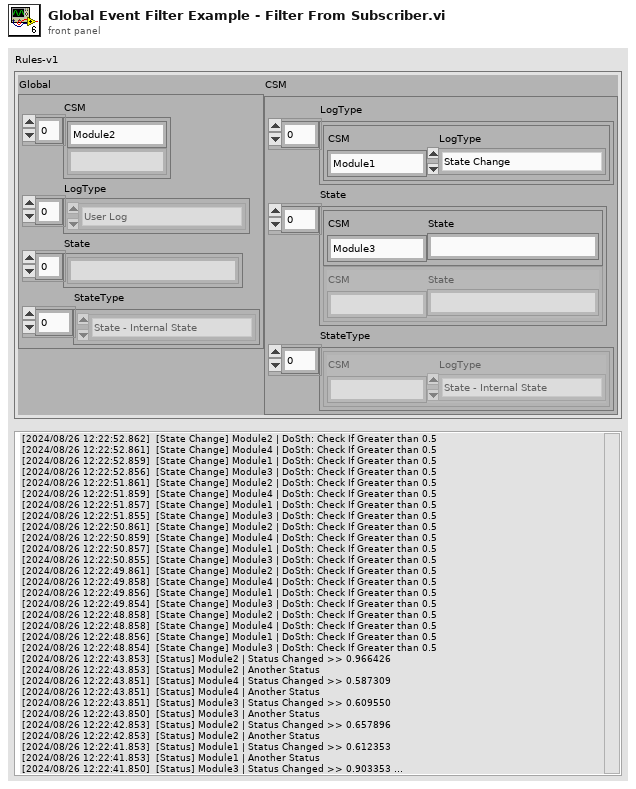
[diagram p1: front panel]
types:
  T1 = typedef "Communicable State Machine.lvlib/_CSM_GlobalLog Filter Rules - v1.0.ctl" = cluster{"Global":cluster{"CSM":string[], "LogType":T2[], "State":string[], "StateType":T3[]}, "CSM":cluster{"LogType":cluster{"CSM":string, "LogType":T2}[], "State":cluster{"CSM":string, "State":string}[], "StateType":cluster{"CSM":string, "LogType":T3}[]}}
  T2 = typedef "Communicable State Machine.lvlib/_CSM_GlobalLog_MSG_TYPE.ctl" = enum16{"User Log", "State Change", "Status", "Interrupt", "Register", "Unregister", "Error Log", "Module Created", "Module Destroyed"}
  T3 = typedef "Communicable State Machine.lvlib/_CSM_GlobalLog_STATE_TYPE.ctl" = enum16{"State - Internal State", "State - External Message", "State - Response", "State - Complete"}
  T4 = typedef "Communicable State Machine.lvlib/_CSM_GlobalLog_MSG.ctl" = cluster{"Name(\"\" to use uuid)":string, "Current State":string, "Arguments":string, "Source Message":T5, "Source Module":string, "Complete(T)/Start(F)":bool, "LogType":T2}
  T5 = typedef "Communicable State Machine.lvlib/_CSM_Response Source Message.ctl" = cluster{"‘State":string, "’Arguments":string, "’Error":errorcluster}
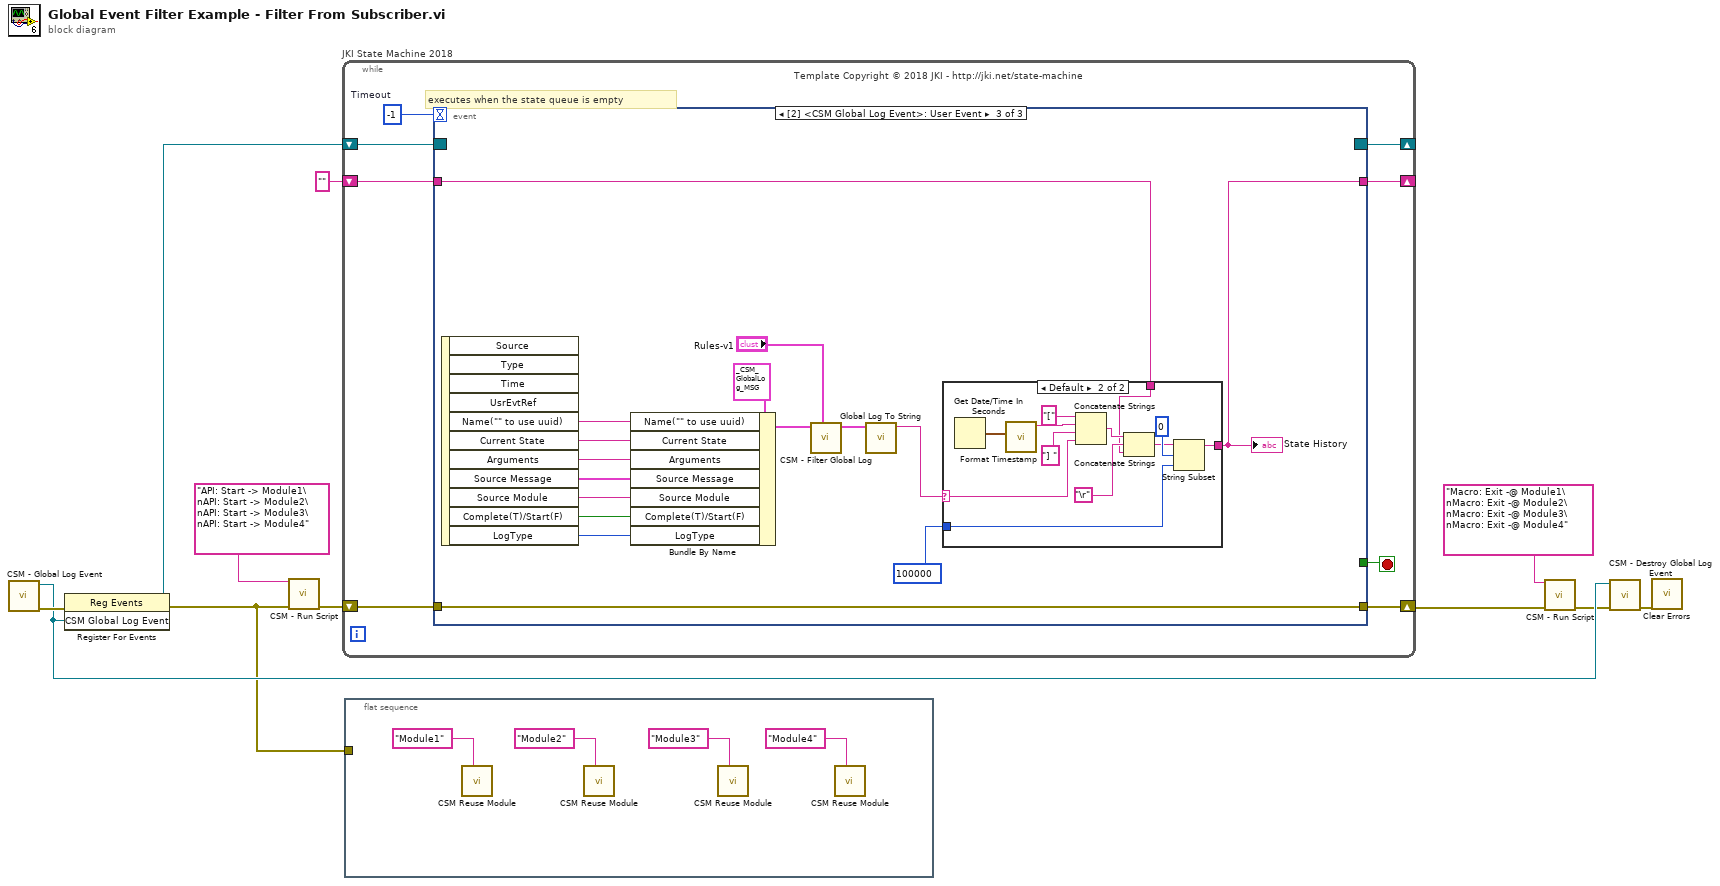
[diagram p0: block diagram]
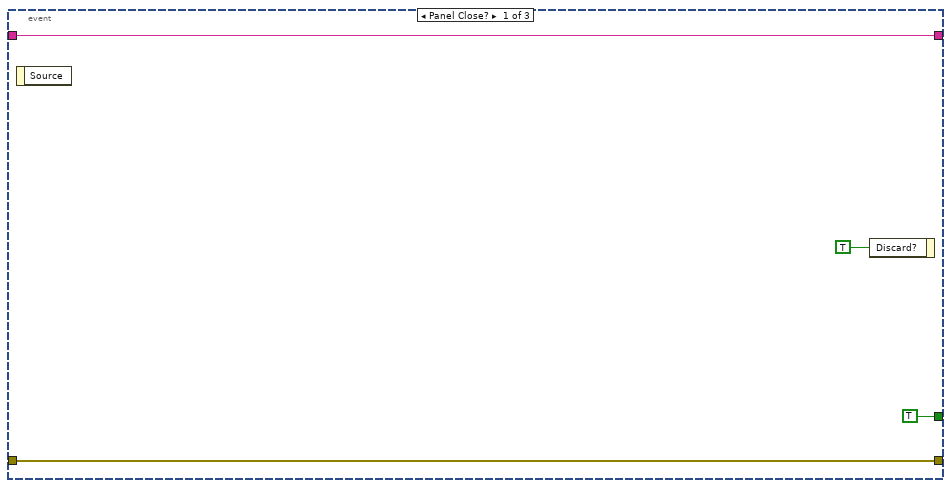
[diagram p2: hidden frame]
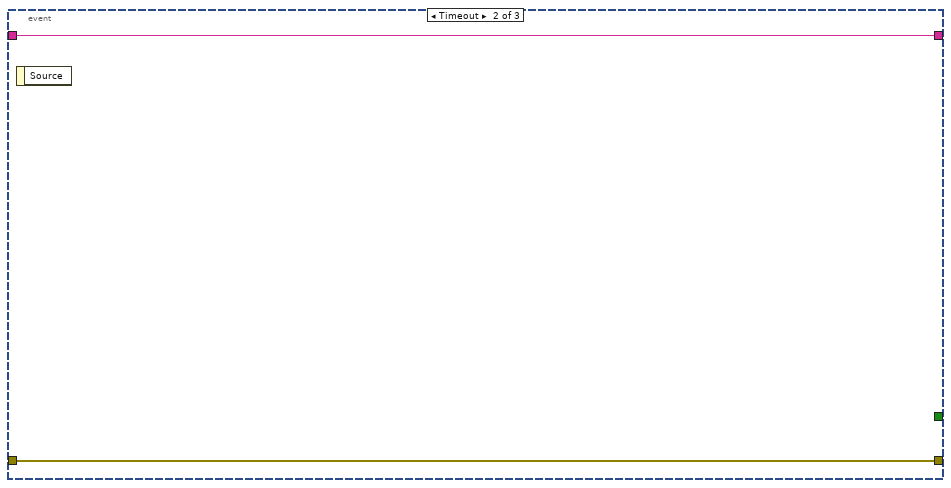
[diagram p3: hidden frame]
diagram:
  n1 = call "CSM - Global Log Event.vi"() -> ("Error out"=w11:errorcluster, "CSM Global Log Event"=w10:refnum<user-event>)  [unwired: 10 in]
  n2 = register-events(error in=w11, w10) -> (reference out=w9:refnum<event-registration>, error out=w1:errorcluster)  [unwired: 1 in]
  n3 = call "CSM - Run Script.vi"("CSM Scripts"="API: Start -> Module1\nAPI: Start -> Module2\nAPI: Start -> Module3\nAPI: Start -> Module4" ("single-line text"), "error in (no error)"=w1) -> ("error out"=w6:errorcluster)  [unwired: 11 in, 2 out]
  n4 = while "JKI State Machine 2018" {
    shift-right: [w19] -> w3
    shift-left: w6 -> [w17]
    shift-right: [w15] -> _
    shift-left: w9 -> [w16]
    shift-right: [w13] -> _
    shift-left: "" -> [w14]
    stop <- w12 stop-if-true
    w18 = -1  # Timeout
    # "executes when the state queue is empty"
    # "Template Copyright © 2018 JKI - http://jki.net/state-machine"
    n5 = event shown="[2] <CSM Global Log Event>: User Event" {
      selector: w16 -> [_ _ _]
      dyn-events: [_ _ _] -> w15
      timeout: w18 -> [_ _ _]
      tunnel: [w23 w25 w41] -> w19
      tunnel: w17 -> [w23 w25 w41]
      tunnel: w14 -> [w21 w24 w30]
      tunnel: [w21 w24 w29] -> w13
      tunnel: [TRUE _ _] -> w12
      event Panel Close? {
        n6 = event-data() -> ()  [unwired: 1 in, 1 out]
        n7 = event-data("Discard?"=TRUE) -> ()  [unwired: 1 in, 1 out]
      }
      event Timeout {
        n8 = event-data() -> ()  [unwired: 1 in, 1 out]
      }
      event User Event {
        n9 = event-data() -> ("Name(\"\" to use uuid)"=w38:string, "Current State"=w37:string, "Arguments"=w36:string, "Source Message"=w35:T5, "Source Module"=w34:string, "Complete(T)/Start(F)"=w33:bool, "LogType"=w32:T2)  [unwired: 1 in, 4 out]
        n10 = Bundle By Name(cluster=T4 {"Name(\"\" to use uuid)"="", "Current State"="", "Arguments"="", "Source Message"={"‘State"="", "’Arguments"="", "’Error"={"status"=FALSE, "code"=0, "source"=""}}, "Source Module"="", "Complete(T)/Start(F)"=FALSE, "LogType"=enum."State Change"} ("Cross CSM Data"), "Name(\"\" to use uuid)"=w38, "Current State"=w37, "Arguments"=w36, "Source Message"=w35, "Source Module"=w34, "Complete(T)/Start(F)"=w33, "LogType"=w32) -> (w28:T4)
        n11 = call-poly "CSM - Filter Global Log.vi"("Rules-v1"="Rules-v1", "Cross CSM Data (in)"=w28) -> ("Cross CSM Data"=w27:T4)  [unwired: 8 in, 1 out]
        n12 = call "Global Log To String.vi"("Log"=w27) -> ("Log String"=w40:string)  [unwired: 9 in]
        n13 = case shown="Default" w40 {
          selector: w40 -> [_ w54]
          tunnel: [w42 w52] -> w29
          tunnel: 100000 ("Toolbar.History Length(char)") -> [_ w51]
          tunnel: w30 -> [w42 w43]
          frame "" {
          }
          frame Default {
            n14 = Get Date/Time In Seconds() -> (seconds since 1Jan1904=w44:timestamp)
            n15 = call "Format Timestamp.vi"("timestamp"=w44) -> ("String"=w45:string)  [unwired: 10 in]
            n16 = Concatenate Strings("[" ("string"), w45, "] " ("string"), w54) -> (w46:string)
            n17 = Concatenate Strings(w46, "\r", w43) -> (w48:string)
            n18 = String Subset(string=w48, offset (0)=0, length (rest)=w51) -> (substring=w52:string)
          }
        }
        "State History" <- w29
      }
    }
  }
  n19 = flat-sequence {
    tunnel: w1 -> [_]
    frame #0 {
      n20 = call "CSM Reuse Module.vi"("Name(\"\" to use uuid)"="Module1" ("Name(\"\" to use uuid)")) -> ()  [unwired: 11 in]
      n21 = call "CSM Reuse Module.vi"("Name(\"\" to use uuid)"="Module2" ("Name(\"\" to use uuid)")) -> ()  [unwired: 11 in]
      n22 = call "CSM Reuse Module.vi"("Name(\"\" to use uuid)"="Module3" ("Name(\"\" to use uuid)")) -> ()  [unwired: 11 in]
      n23 = call "CSM Reuse Module.vi"("Name(\"\" to use uuid)"="Module4" ("Name(\"\" to use uuid)")) -> ()  [unwired: 11 in]
    }
  }
  n24 = call "CSM - Run Script.vi"("CSM Scripts"="Macro: Exit -@ Module1\nMacro: Exit -@ Module2\nMacro: Exit -@ Module3\nMacro: Exit -@ Module4" ("single-line text"), "error in (no error)"=w3) -> ("error out"=w2:errorcluster)  [unwired: 11 in, 2 out]
  n25 = call "CSM - Destroy Global Log Event.vi"("Error in"=w2, "CSM Global Log Event"=w10) -> ("Error out"=w8:errorcluster)  [unwired: 9 in]
  n26 = call <vilib>:"Clear Errors.vi"("error in (no error)"=w8) -> ()  [unwired: 5 in, 2 out]
